vi "Save As FITS.vi"(8 "error in (no error)":errorcluster, 10 "typ":i32, 11 "szFileTitle":string) -> (0 "error out":errorcluster, 2 "function return":u32, 3 "szFileTitle out":string)   [LabVIEW 2018, in "AndorSDK.lvlib"]
doc: "EXPNETTYPE unsigned int WINAPI SaveAsFITS(char * szFileTitle, int typ);"
uses:
  AndorSDK.lvlib
  ATMCD32D.dll
  OwnVIs/AndorOWN.lvlib
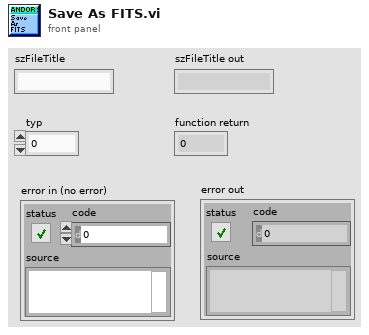
[diagram p1: front panel]
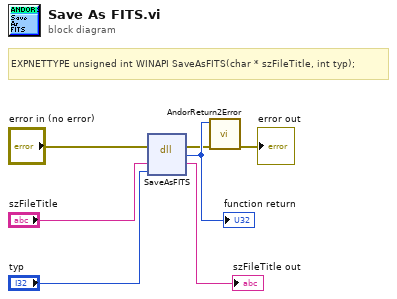
[diagram p0: block diagram]
diagram:
  # "EXPNETTYPE unsigned int WINAPI SaveAsFITS(char * szFileTitle, int typ);"
  n1 = dll-call lib="C:/Users/johan/Downloads/LabVIEW software/LabVIEW software/IX-81 Software/lib/ANDOR/Andor SDK/ATMCD32D.*" fn="SaveAsFITS"(error in="error in (no error)", "szFileTitle"="szFileTitle", "typ"="typ") -> (error out=w2:errorcluster, w3:u32, "szFileTitle"=→"szFileTitle out":string)  [unwired: 3 in, 1 out]
  "function return" <- w3
  n2 = call "AndorReturn2Error.vi"("error in (no error)"=w2, "Camera return"=w3) -> ("error out"=→"error out":errorcluster)  [unwired: 9 in]
